vi "Globals.vi"() -> ()   [LabVIEW 2012]
panel:
  in  "IR Block":dbl
  in  "Robot Velocities":T1
  in  "IR Right":dbl
  in  "IR Left":dbl
  in  "IR Front":dbl
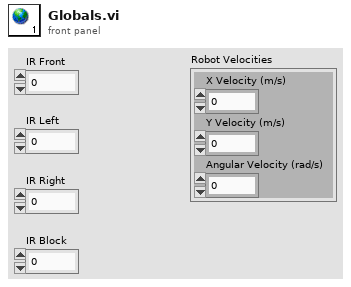
[diagram p1: front panel]
types:
  T1 = cluster{"X Velocity (m/s)":dbl, "Y Velocity (m/s)":dbl, "Angular Velocity (rad/s)":dbl}
diagram:
